vi "Clear Fault.vi"(8 "error in":errorcluster, 9 "timeout (-1)":i32=-1, 10 "code":i32, 11 "Engine Runtime Interface in":refnum<class "Engine Runtime Interface.lvclass">) -> (0 "error out":errorcluster, 3 "Engine Runtime Interface out":refnum<class "Engine Runtime Interface.lvclass">)   [LabVIEW 2013, in "Engine Runtime Interface.lvclass"]
doc: "Clears the record of a fault in the engine."
uses:
  Engine Runtime Interface.lvclass
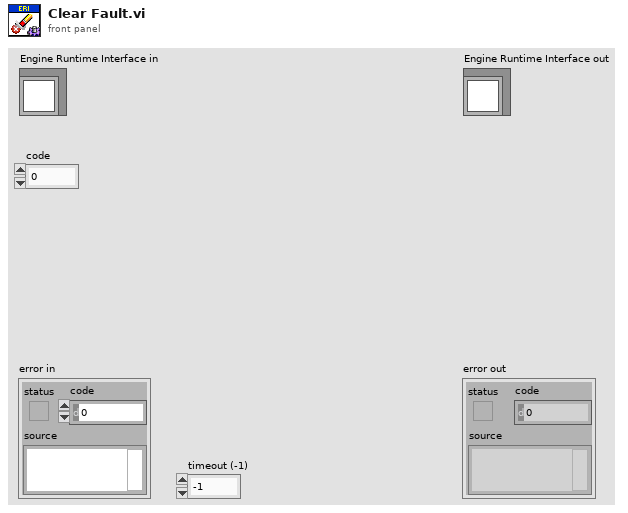
[diagram p1: front panel]
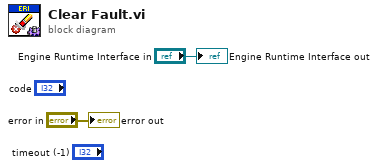
[diagram p0: block diagram]
diagram:
  "error out" <- "error in"
  "Engine Runtime Interface out" <- "Engine Runtime Interface in"
